vi "Check Min-Max.vi"(8 "error in (no error)":errorcluster, 11 "Numeric Data Type in":refnum<class "Numeric Data Type.lvclass">) -> (0 "error out":errorcluster, 3 "Numeric Data Type (dup)":refnum<class "Numeric Data Type.lvclass">)   [LabVIEW 2018, in "Numeric Data Type.lvclass"]
uses:
  Numeric Data Type.lvclass
  Numeric Data Type.lvclass/Numeric Data Type.ctl
  Reference Min-Max Warning.vi
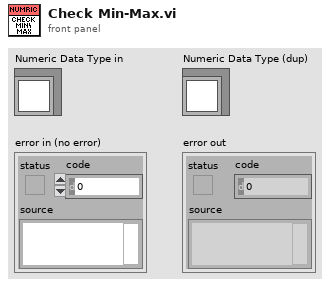
[diagram p1: front panel]
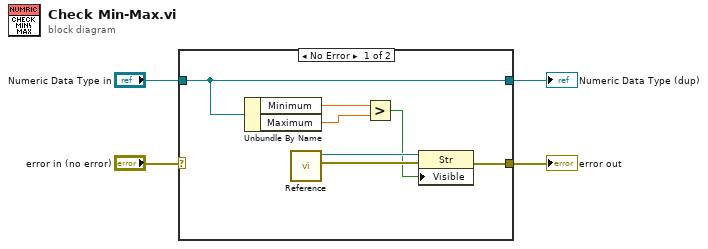
[diagram p0: block diagram]
diagram:
  n1 = case shown="No Error" "error in (no error)" {
    selector: "error in (no error)" -> [_ w13]
    tunnel: [w5 w13] -> w3
    tunnel: [w11 w12] -> w1
    tunnel: "Numeric Data Type in" -> [w11 w12]
    frame No Error {
      n2 = Unbundle By Name(w11) -> ("Minimum"=w9:dbl, "Maximum"=w10:dbl)
      n3 = call-poly "Reference.vi"() -> ("error out"=w7:errorcluster, "Min/Max Warning"=w8:refnum<vi>)  [unwired: 10 in]
      n4 = Greater?(x=w9, y=w10) -> (0:w6:bool)
      n5 = property class="Str"(reference=w8, error in=w7, "Visible"=w6) -> (error out=w5:errorcluster)  [unwired: 1 out]
    }
    frame Error {
    }
  }
  "error out" <- w3
  "Numeric Data Type (dup)" <- w1
